vi "setframerate.vi"(8 "error in (no error)":errorcluster, 11 "Imaging in":refnum<class "Imaging.lvclass">) -> (0 "error out":errorcluster, 3 "Imaging out":refnum<class "Imaging.lvclass">)   [LabVIEW 2014, in "Imaging.lvclass"]
uses:
  Imaging.lvclass
  <resource>/objmgr/imaqdx.rc
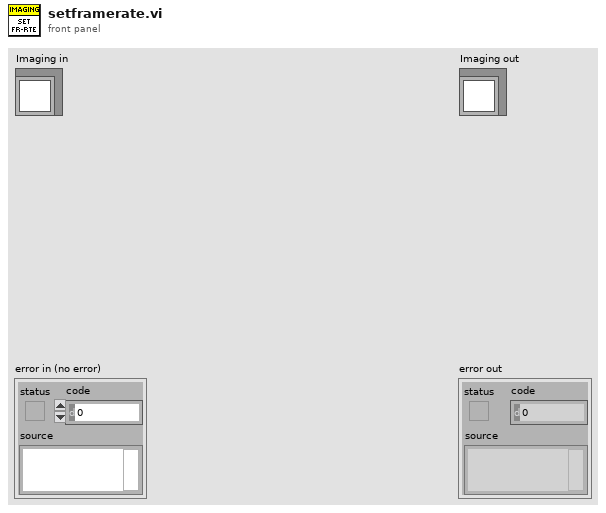
[diagram p1: front panel]
types:
  T1 = typedef "IMAQdx.ctl" = refnum<k21>
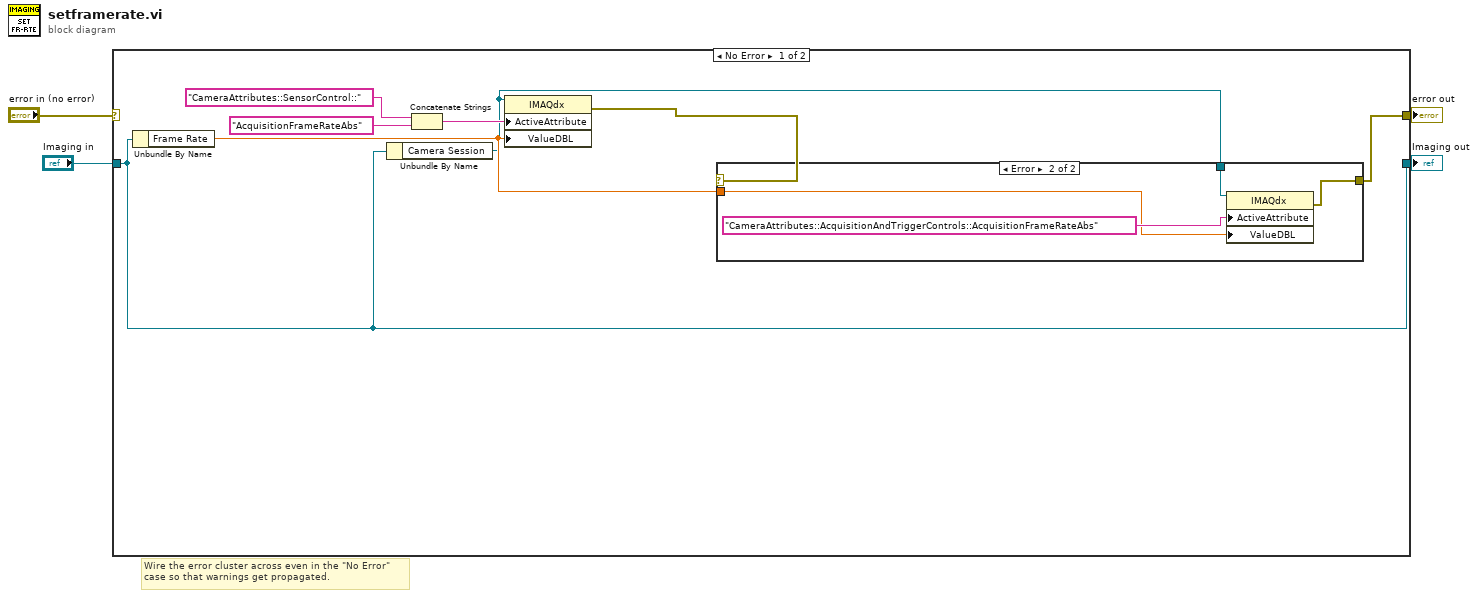
[diagram p0: block diagram]
diagram:
  # "Wire the error cluster across even in the \"No Error\"\ncase so that warnings get propagated."
  n1 = case shown="No Error" "error in (no error)" {
    selector: "error in (no error)" -> [_ w19]
    tunnel: [w6 w19] -> w3
    tunnel: [w9 w18] -> w1
    tunnel: "Imaging in" -> [w9 w18]
    frame No Error {
      n2 = Unbundle By Name(w9) -> ("Frame Rate"=w7:dbl)
      n3 = Unbundle By Name(w9) -> ("Camera Session"=w5:T1)
      n4 = Concatenate Strings("CameraAttributes::SensorControl::" ("string"), "AcquisitionFrameRateAbs" ("string")) -> (w10:string)
      n5 = property class="IMAQdx"(reference=w5, "ActiveAttribute"=w10, "ValueDBL"=w7) -> (error out=w8:errorcluster)  [unwired: 1 in, 1 out]
      n6 = case shown="Error" w8 {
        selector: w8 -> [w13 _]
        tunnel: w7 -> [_ w16]
        tunnel: [w13 w15] -> w6
        tunnel: w5 -> [_ w14]
        frame No Error {
        }
        frame Error {
          n7 = property class="IMAQdx"(reference=w14, "ActiveAttribute"="CameraAttributes::AcquisitionAndTriggerControls::AcquisitionFrameRateAbs" ("string"), "ValueDBL"=w16) -> (error out=w15:errorcluster)  [unwired: 1 in, 1 out]
        }
      }
    }
    frame Error {
    }
  }
  "error out" <- w3
  "Imaging out" <- w1
